vi "Select_data_set.vi"(2 "array":dbl[][][](array[numeric]), 3 "index":i32) -> (0 "Array 2":dbl[][](array[numeric]))   [LabVIEW 2015]
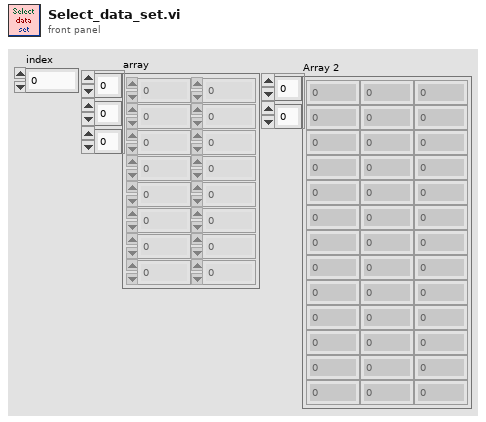
[diagram p1: front panel]
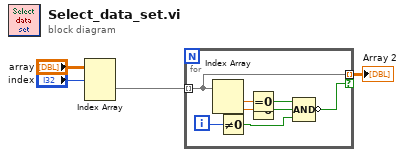
[diagram p0: block diagram]
diagram:
  n1 = Index Array(array="array", index (dim 0)="index") -> (element=w2:dbl[][])  [unwired: 2 in]
  n2 = for {
    tunnel: w2 -> [w12] mode=indexing
    tunnel: [w12] -> w4 mode=indexing if=w5
    i -> [w11]
    n3 = Index Array(array=w12) -> (element #1=w9:dbl, element #2=w8:dbl)  [unwired: 2 in]
    n4 = Not Equal To 0?(x=w11) -> (x != 0?=w6:bool)
    n5 = Equal To 0?(x=w9) -> (x = 0?=w10:bool)
    n6 = Equal To 0?(x=w8) -> (x = 0?=w7:bool)
    n7 = Compound Arithmetic op=AND(w10, w7, w6) -> (invert w5:bool)
  }
  "Array 2" <- w4
